vi "Read Engine.vi"(8 "error in (no error)":errorcluster, 11 "ContextData in":refnum<class "ContextData.lvclass">) -> (0 "error out":errorcluster, 2 "Simon_Engine.lvclass":refnum<class "Simon_Engine.lvclass">, 3 "ContextData out":refnum<class "ContextData.lvclass">)   [LabVIEW 2019, in "ContextData.lvclass"]
uses:
  ContextData.lvclass
  Simon_Engine/Simon_Engine.lvclass
  ContextData.lvclass/ContextData.ctl
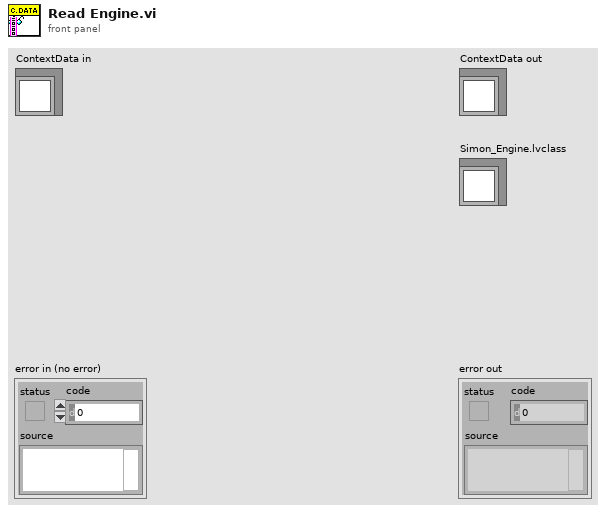
[diagram p1: front panel]
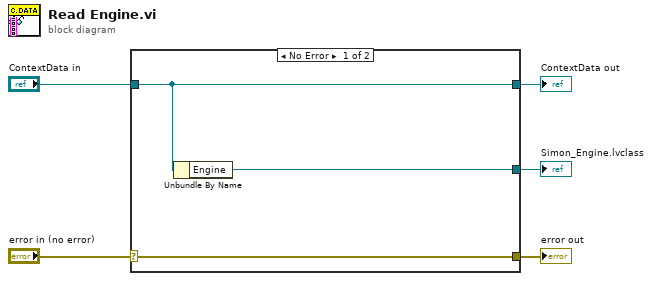
[diagram p0: block diagram]
diagram:
  n1 = case shown="No Error" "error in (no error)" {
    selector: "error in (no error)" -> [w8 w9]
    tunnel: [w8 w9] -> w4
    tunnel: [w7 w10] -> w2
    tunnel: "ContextData in" -> [w7 w10]
    tunnel: [w6 _] -> w1
    frame No Error {
      n2 = Unbundle By Name(w7) -> ("Engine"=w6:refnum<class "Simon_Engine.lvclass">)
    }
    frame Error {
    }
  }
  "error out" <- w4
  "ContextData out" <- w2
  "Simon_Engine.lvclass" <- w1
